vi "Sort Palette Items.vi"(1 "Array 2":T1[](array[typedef])) -> (0 "Array":T1[](array[typedef]))   [LabVIEW 2018, in "Palette Generation.lvlib"]
uses:
  Palette Generation.lvlib
  <vilib>/Palette API/Palette Menu/Public Type Define/Item.ctl
  <vilib>/Palette API/Palette Menu/Palette Menu.lvlib
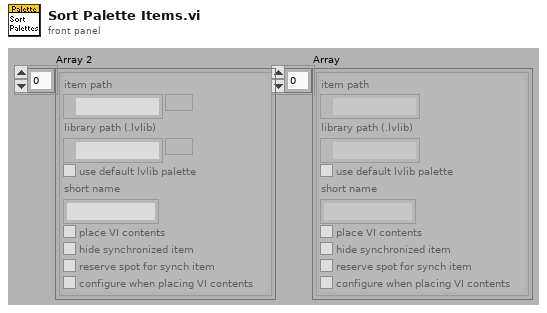
[diagram p1: front panel]
types:
  T1 = typedef "Palette Menu.lvlib/Item.ctl" = cluster{"item path":path, "library path (.lvlib)":path, "use default lvlib palette":bool, "short name":string, "place VI contents":bool, "hide synchronized item":bool, "reserve spot for synch item":bool, "configure when placing VI contents":bool}
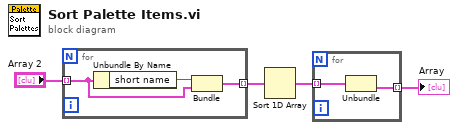
[diagram p0: block diagram]
diagram:
  n1 = for {
    tunnel: "Array 2" -> [w6] mode=indexing
    tunnel: [w5] -> w1 mode=indexing
    n2 = Unbundle By Name(w6) -> ("short name"=w7:string)
    n3 = Bundle("short name"=w7, "Items"=w6) -> (w5:cluster{"short name":string, "Items":T1})  [unwired: 1 out]
  }
  n4 = Sort 1D Array(array=w1) -> (sorted array=w2:cluster{"short name":string, "Items":T1}[])
  n5 = for {
    tunnel: w2 -> [w9] mode=indexing
    tunnel: [w8] -> w4 mode=indexing
    n6 = Unbundle(w9) -> ("Items"=w8:T1)  [unwired: 1 out]
  }
  "Array" <- w4
